vi "ProcesadorDTMFSignalsV1.vi"() -> ()   [LabVIEW 2020]
uses:
  <vilib>/express/express analysis/Spectral/XNode/ExpressSpectralMeasurementsBlockNode.xnode
  <vilib>/express/express analysis/Spectral/Block/exnSpectralBlock spectral measurements peak poly.vi
  <vilib>/express/express analysis/Spectral/Block/exnSpectralBlock spectral measurements peak DDT.vi
  <vilib>/measure/NI_MAPro.lvlib
  <vilib>/measure/matone.llb/Extract Multiple Tone Information N Chan.vi
panel:
  in  "Min_Frecuencias":dbl[](array[numeric])=[697.0, 770.0, 852.0, 941.0]
  in  "Max_Frecuencias":dbl[](array[numeric])=[1209.0, 1336.0, 1477.0, 1633.0]
  in  "stop":bool
  out "Waveform Graph":dynamicdata(graph)
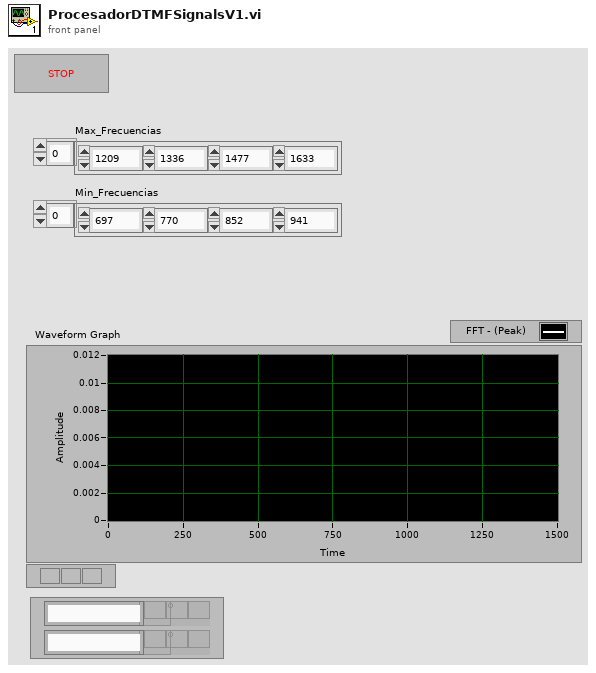
[diagram p1: front panel]
types:
  T1 = cluster{"averaging mode":u16, "weighting mode":u16, "number of averages":u32}
  T2 = cluster{"dB On (F)":bool, "unwrap phase (F)":bool, "convert to degree (F)":bool}
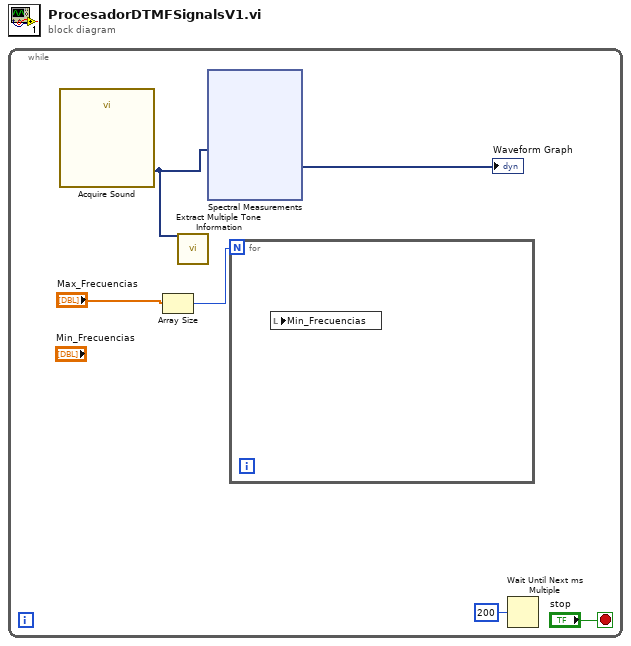
[diagram p0: block diagram]
diagram:
  n1 = while {
    stop <- "stop" stop-if-true
    n2 = call "Acquire Sound"() -> ("Data"=w3:dynamicdata)  [unwired: 18 in, 1 out]
    n3 = Array Size(array="Max_Frecuencias") -> (size(s)=w1:i32)
    n4 = call-poly <vilib>:"Extract Multiple Tone Information.vi"("time signals in"=w3) -> ()  [unwired: 12 in, 3 out]
    n5 = xnode "Spectral Measurements"("Signals"=w3) -> ("FFT - (Peak)"=→"Waveform Graph":dynamicdata)  [unwired: 1 in, 2 out]
    n6 = for {
      N: w1 -> [_]
      n7 = local read "Min_Frecuencias"() -> ()  [unwired: 1 in]
    }
    n8 = Wait Until Next ms Multiple(millisecond multiple=u32 200) -> ()  [unwired: 1 out]
  }
